vi "PH_Sixpack.SetPeakCurrent.vi"(0 "i ref in":refnum<vi>, 1 "MotNr (0+1)":enum8{"0+1", "2+3", "4+5"}(ring)=enum."4+5", 4 "Device Error in":errorcluster, 5 "error in":errorcluster) -> (14 "i ref out":refnum<vi>, 16 "ok?":bool, 18 "Device Error out":errorcluster, 19 "error out":errorcluster)   [LabVIEW 2014, in "PH_Sixpack.lvlib"]
doc: "This VI acts on the hardware."
uses:
  PH_Sixpack.lvlib
  instr.lib/SixPack/Sixpack - Driver.lvlib
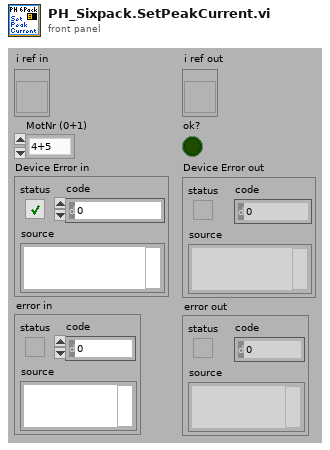
[diagram p1: front panel]
types:
  T1 = typedef "PH_Sixpack.lvlib/PH_Sixpack.Axis Cluster.ctl" = cluster{"Config":T2, "To set?":cluster{"VmaxAmax":bool, "I max":bool, "VStartVminDivi":bool, "Ref Search Parameter":bool, "Stopswitch Limits":bool, "Axis Parameter":bool, "I Control":bool}}
  T2 = typedef "PH_Sixpack.lvlib/PH_Sixpack.Axis Configuration.ctl" = cluster{"VmaxAmax":T3, "I max (50%)":T4, "VStartVminDivi":T5, "Ref Search Parameter":T6, "Stopswitch Limits":T7, "Axis Parameter":T8, "I Control":T11}
  T3 = typedef "Sixpack - Driver.lvlib/VmaxAmax.ctl" = cluster{"VMax(511)":u16, "AMax(128)":u16}
  T4 = typedef "Sixpack - Driver.lvlib/PeakCurrent.ctl" = dbl
  T5 = typedef "Sixpack - Driver.lvlib/VStartVmin.ctl" = cluster{"VStart(5)":u16, "Vmin(4)":u16, "Div i (2)":enum8{"0", "1", "2", "3"}}
  T6 = typedef "Sixpack - Driver.lvlib/Ref Search Parameter.ctl" = cluster{"VRefMax(100)":u16, "DebouncingTime (22ms)":u8}
  T7 = typedef "Sixpack - Driver.lvlib/Stopswitch Limits.ctl" = cluster{"MinLeft(0)":u16, "MaxRight(1023)":u16}
  T8 = typedef "Sixpack - Driver.lvlib/Motor Parameter.ctl" = cluster{"Poslimit (6400)":u32, "P5 Bits":T9, "P6 Bits":T10}
  T9 = typedef "Sixpack - Driver.lvlib/MotorParameter_P5.ctl" = cluster{"MT_PI":bool, "MT_ROTARY":bool, "MT_AUTONULLCMD":bool, "MT_TESTNULL":bool, "MT_NULLLEFT":bool, "MT_NULLCENTRE":bool, "MT_STOPNULL":bool, "MT_FILTERSWITCH":bool}
  T10 = typedef "Sixpack - Driver.lvlib/MotorParameter_P6.ctl" = cluster{"MT_OPTIMIZEWAY":bool, "MT_FASTREF":bool, "MT_MECHREF":bool, "MT_DELAYTESTNULL":bool, "MT_STOPSOFT":bool, "MT_STOPNOREF":bool, "MT_NULLPOSITIVE":bool, "MUT_STOPFULSTEPS":bool}
  T11 = typedef "Sixpack - Driver.lvlib/Current Control.ctl" = cluster{"PowerDownDelay (500)":u16, "PowerDown (0%)":T12, "Standing (50%)":T12, "Running (75%)":T12, "Accelerating (100%)":T12}
  T12 = typedef "Sixpack - Driver.lvlib/Current.ctl" = enum8{"100%", "75%", "50%", "38%", "25%", "19%", "13%", "9%", "0%"}
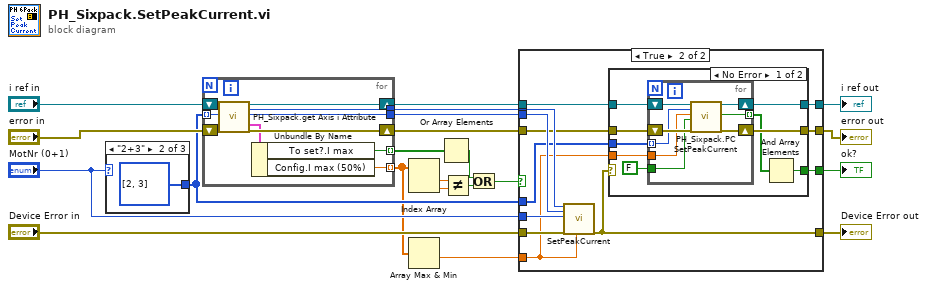
[diagram p0: block diagram]
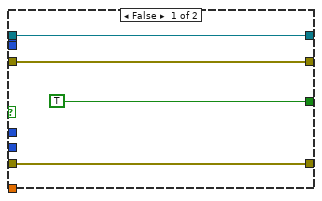
[diagram p2: hidden frame]
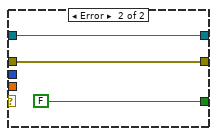
[diagram p3: hidden frame]
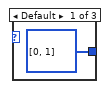
[diagram p4: hidden frame]
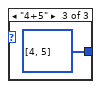
[diagram p5: hidden frame]
diagram:
  n1 = case shown="\"2+3\"" "MotNr (0+1)" {
    tunnel: [i32[] [0, 1] i32[] [2, 3] i32[] [4, 5]] -> w9
    frame Default {
    }
    frame "2+3" {
    }
    frame "4+5" {
    }
  }
  n2 = for {
    tunnel: [w32] -> w18
    tunnel: [w31] -> w17
    shift-right: [w34] -> w15
    shift-left: "i ref in" -> [w25]
    shift-right: [w33] -> w13
    shift-left: "error in" -> [w26]
    tunnel: [w27] -> w6 mode=indexing
    tunnel: w9 -> [w28] mode=indexing
    tunnel: [w29] -> w7 mode=indexing
    n3 = call "PH_Sixpack.get Axis i Attribute.vi"("VI in"=w25, "Axis"=w28, "error in"=w26) -> ("VI out"=w34:refnum<vi>, "HANDLE"=w32:i32, "SixPack ID(0)"=w31:u16, "Axis Attributes"=w30:T1, "error out"=w33:errorcluster)  [unwired: 10 in, 2 out]
    n4 = Unbundle By Name(w30) -> ("To set?.I max"=w29:bool, "Config.I max (50%)"=w27:T4)
  }
  n5 = Index Array(array=w6) -> (element #1=w5:T4, element #2=w4:T4)  [unwired: 2 in]
  n6 = Array Max & Min(array=w6) -> (min value=w10:T4)  [unwired: 3 out]
  n7 = Or Array Elements(Boolean array=w7) -> (logical OR=w1:bool)
  n8 = Not Equal?(x=w5, y=w4) -> (x != y?=w2:bool)
  n9 = Or(x=w1, y=w2) -> (x .or. y?=w3:bool)
  n10 = case shown="True" w3 {
    tunnel: "Device Error in" -> [w35 w50]
    tunnel: w18 -> [_ w49]
    tunnel: w17 -> [_ w48]
    tunnel: "MotNr (0+1)" -> [_ w47]
    tunnel: w15 -> [w38 w46]
    tunnel: [w38 w45] -> w14
    tunnel: w13 -> [w37 w44]
    tunnel: [w37 w43] -> w12
    tunnel: [w35 w42] -> w11
    tunnel: w10 -> [_ w39]
    tunnel: w9 -> [_ w41]
    tunnel: [TRUE w40] -> w8
    frame False {
    }
    frame True {
      n11 = call "SetPeakCurrent.vi"("handle in"=w49, "UnitAddress (0)"=w48, "MotNr (0+1)"=w47, "error in(no error)"=w50, "Imax (50%)"=w39) -> ("error out"=w42:errorcluster)  [unwired: 13 in, 1 out]
      n12 = case shown="No Error" w42 {
        tunnel: w44 -> [w59 w69]
        tunnel: [w56 w69] -> w43
        tunnel: w46 -> [w58 w70]
        tunnel: [w57 w70] -> w45
        tunnel: w41 -> [w54 _]
        tunnel: w39 -> [w53 _]
        tunnel: [w51 FALSE] -> w40
        frame No Error {
          n13 = for {
            tunnel: w54 -> [w62] mode=indexing
            tunnel: w53 -> [w61]
            shift-right: [w64] -> w56
            shift-left: w59 -> [w67]
            shift-right: [w65] -> w57
            shift-left: w58 -> [w66]
            tunnel: FALSE ("To set?") -> [w60]
            tunnel: [w63] -> w55 mode=indexing
            n14 = call "PH_Sixpack.PC SetPeakCurrent.vi"("i ref in"=w66, "Axis"=w62, "Imax (50%)"=w61, "To set?"=w60, "error in"=w67) -> ("i ref out"=w65:refnum<vi>, "ok?"=w63:bool, "error out"=w64:errorcluster)  [unwired: 12 in]
          }
          n15 = And Array Elements(Boolean array=w55) -> (logical AND=w51:bool)
        }
        frame Error {
        }
      }
    }
  }
  "error out" <- w12
  "i ref out" <- w14
  "Device Error out" <- w11
  "ok?" <- w8
